vi "Tester_VI.vi"() -> ()   [LabVIEW 2021]
doc: "This VI Rolls over the Voltage range and determine the Fault point at which the Module fails."
uses:
  Assignment 1/Assign 2/Input cluster.ctl
panel:
  in  "Cluster":T1={"Resolution[V]"=0.01, "Maximum[V]"=5.0, "Minimum[V]"=3.0} {"Minimum[V]" step=0.01 format="%#.2g"; "Maximum[V]" step=0.01 format="%#.2g"; "Resolution[V]" min=1e-06 max=1.0 step=0.01}
  in  "Stop":bool
  out "Voltage_Failure_Point(V)":dbl format="%#.8g"
  # "FAULT POINT TESTER"
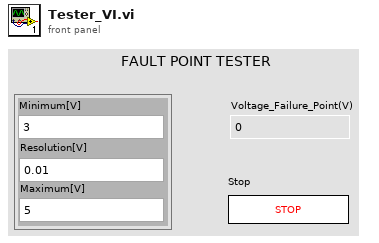
[diagram p1: front panel]
types:
  T1 = typedef "Input cluster.ctl" = cluster{"Resolution[V]":dbl, "Maximum[V]":dbl, "Minimum[V]":dbl}
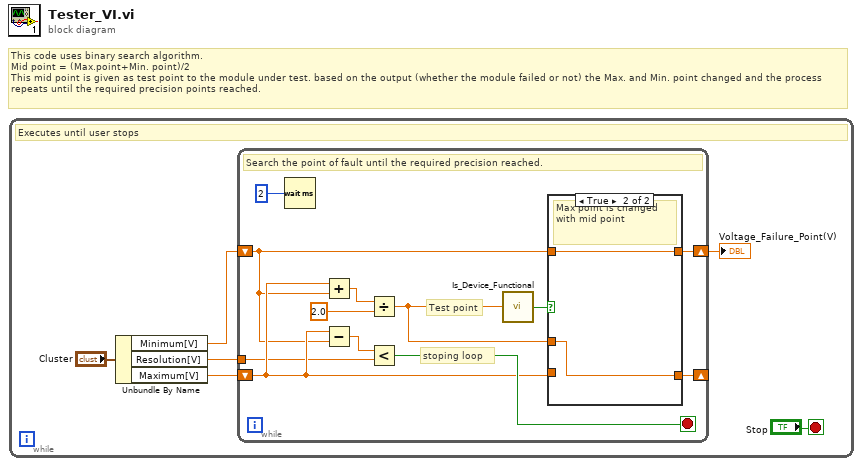
[diagram p0: block diagram]
diagram:
  # "This code uses binary search algorithm.\nMid point = (Max.point+Min. point)/2\nThis mid point is given as test point to the module under test. based on the output (whether the module failed or not) the Max. and Min. point changed and the process repeats until the required precision points reached."
  n1 = while {
    stop <- "Stop" stop-if-true
    # "Executes until user stops"
    n2 = Unbundle By Name("Cluster") -> ("Minimum[V]"=w3:dbl, "Resolution[V]"=w2:dbl, "Maximum[V]"=w1:dbl)
    n3 = while {
      shift-right: [w16] -> w6
      shift-left: w3 -> [w8]
      shift-right: [w15] -> _
      shift-left: w1 -> [w12]
      tunnel: w2 -> [w11]
      stop <- w14 stop-if-true
      # "stoping loop"
      # "Test point"
      # "Search the point of fault until the required precision reached."
      n4 = Wait (ms)(milliseconds to wait=u32 2) -> ()  [unwired: 1 out]
      n5 = Add(x=w12, y=w8) -> (x+y=w18:dbl)
      n6 = Subtract(x=w12, y=w8) -> (x-y=w13:dbl)
      n7 = Divide(x=w18, y=2.0) -> (x/y=w9:dbl)
      n8 = Less?(x=w13, y=w11) -> (x < y?=w14:bool)
      n9 = call "Is_Device_Functional.vi"("Operating_Voltage(V)"=w9) -> ("Device_Functional"=w10:bool)  [unwired: 14 in]
      n10 = case shown="True" w10 {
        tunnel: w8 -> [_ w21]
        tunnel: w12 -> [w19 _]
        tunnel: w9 -> [w20 w22]
        tunnel: [w20 w21] -> w16
        tunnel: [w19 w22] -> w15
        frame False {
          # "Min point is changed with mid point"
        }
        frame True {
          # "Max point is changed with mid point"
        }
      }
    }
    "Voltage_Failure_Point(V)" <- w6
  }
